vi "Add to Compressed File.vi"(8 "error in (no error)":errorcluster, 9 "File or Folder to be compressed":path, 10 "Compressed File Path":path, 11 "7-zip Wrapper in":refnum<class "7-zip Wrapper.lvclass">) -> (0 "error out":errorcluster, 3 "7-zip Wrapper out":refnum<class "7-zip Wrapper.lvclass">)   [LabVIEW 2020, in "7-zip Wrapper.lvclass"]
uses:
  7-zip Wrapper.lvclass
  C:/Users/fflores/Documents/GitHub Projects/LabVIEW-CLI-Wrapper/Console Wrapper/Console Wrapper.lvclass
  Console Wrapper/Console Wrapper.lvclass/Console Wrapper.ctl
  Console Wrapper/Write Command Options.vi
  Console Wrapper/Write Command.vi
  Console Wrapper/Console Wrapper.lvclass
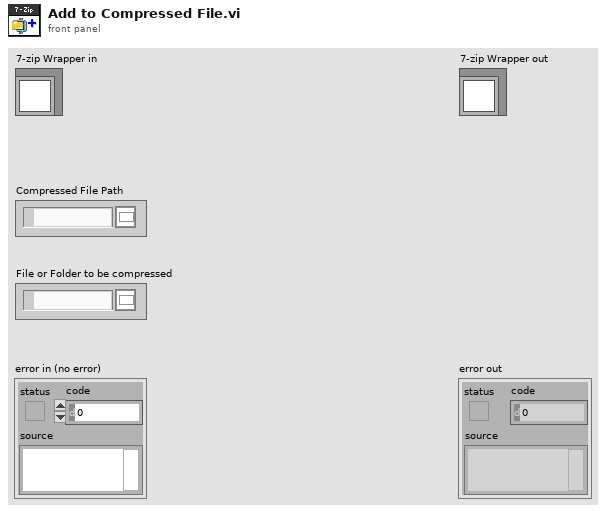
[diagram p1: front panel]
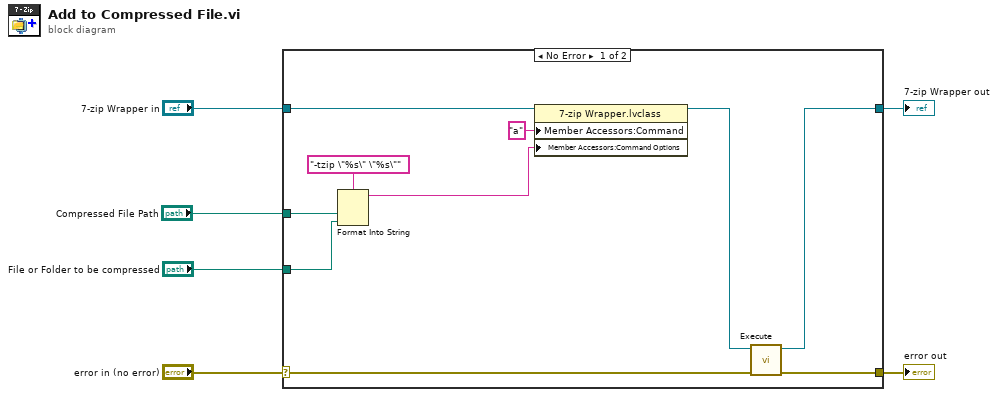
[diagram p0: block diagram]
diagram:
  n1 = case shown="No Error" "error in (no error)" {
    selector: "error in (no error)" -> [w16 w18]
    tunnel: [w15 w18] -> w5
    tunnel: [w13 w17] -> w3
    tunnel: "7-zip Wrapper in" -> [w14 w17]
    tunnel: "Compressed File Path" -> [w10 _]
    tunnel: "File or Folder to be compressed" -> [w9 _]
    frame No Error {
      n2 = Format Into String(format string="-tzip \"%s\" \"%s\"", w10, w9) -> (resulting string=w7:string)  [unwired: 2 in, 1 out]
      n3 = property class="7-zip Wrapper.lvclass"(reference=w14, "Member Accessors:Command"="a" ("Command"), "Member Accessors:Command Options"=w7) -> (reference out=w12:refnum<class "7-zip Wrapper.lvclass">)  [unwired: 1 in, 1 out]
      n4 = call "Execute.vi"("error in (no error)"=w16, "Console Wrapper in"=w12) -> ("error out"=w15:errorcluster, "Console Wrapper out"=w13:refnum<class "7-zip Wrapper.lvclass">)  [unwired: 7 in, 1 out]
    }
    frame Error {
    }
  }
  "error out" <- w5
  "7-zip Wrapper out" <- w3
